vi "KG set total flow sp.vi"(8 "Fehler (Eingang, kein Fehler)":errorcluster, 10 "total flow setpoint":dbl, 11 "VISA-Ressourcenname":refnum<visa-resource-name>) -> (0 "Fehler (Ausgang)":errorcluster, 2 "Kommando gesendet":string, 3 "VISA-Ressourcenname (Ausgang)":refnum<visa-resource-name>)   [LabVIEW 2020, in "Linearisierung v2.lvlib" / "Gasteiler.lvlib" / "HovaCAL_Interface.lvlib" / "KGN.lvlib" / "set.lvlib"]
uses:
  set.lvlib
  KGN.lvlib
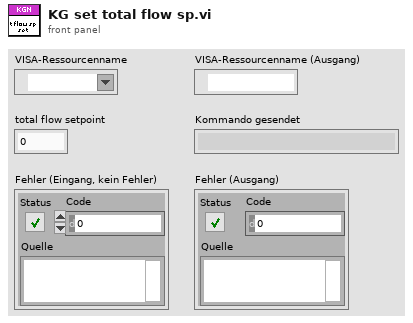
[diagram p1: front panel]
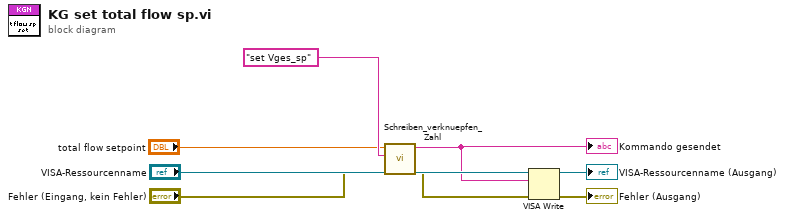
[diagram p0: block diagram]
diagram:
  n1 = call "Schreiben_verknuepfen_Zahl.vi"("error in (no error)"="Fehler (Eingang, kein Fehler)", "Order"="set Vges_sp" ("Schreibpuffer"), "Zahl"="total flow setpoint") -> ("error out"=w1:errorcluster, "Verknüpfter String"=w4:string)  [unwired: 7 in]
  "Kommando gesendet" <- w4
  n2 = VISA Write(VISA resource name="VISA-Ressourcenname", write buffer=w4, error in (no error)=w1) -> (VISA resource name out=→"VISA-Ressourcenname (Ausgang)":refnum<visa-resource-name>, error out=→"Fehler (Ausgang)":errorcluster)  [unwired: 1 out]
